vi "QCPFileWrite.vi"(9 "Path Relative?":bool=TRUE, 10 "File Path":string, 11 "QCP Data Block In":T1) -> (0 "error out":errorcluster, 3 "QCP Data Block Out":T1)   [LabVIEW 2015]
uses:
  <userlib>/836-Library/System/QCP Support Code/QCP Data Block.ctl
  <vilib>/Utility/file.llb/Write To Spreadsheet File (string).vi
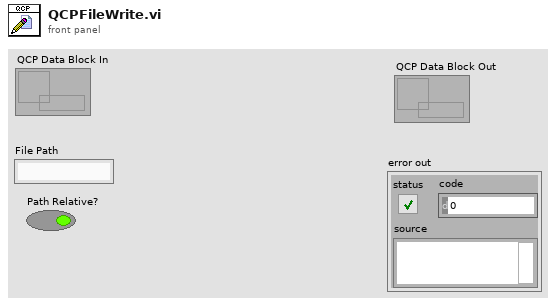
[diagram p1: front panel]
types:
  T1 = typedef "QCP Data Block.ctl" = refnum<data-value>
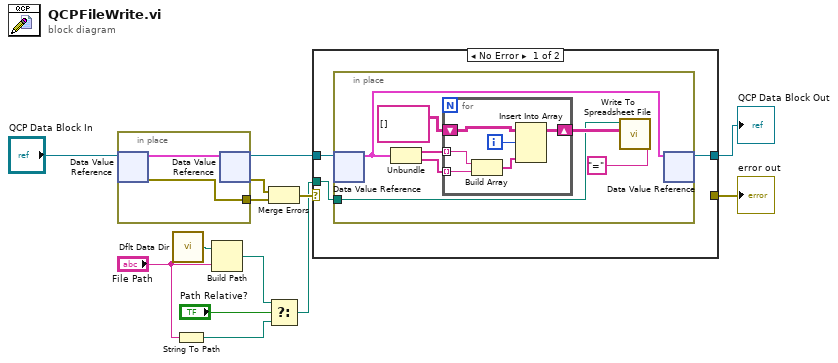
[diagram p0: block diagram]
diagram:
  n1 = in-place {
    in-place-border: [w14] -> w12
    n2 = in-place-dvr #1("QCP Data Block In") -> (w15:cluster{string[], string[]}, w14:errorcluster)
    n3 = in-place-dvr #1(w15) -> (w10:T1, w13:errorcluster)
  }
  n4 = call <vilib>:"Dflt Data Dir.vi"() -> ("App:Default Data Directory"=w1:path)
  n5 = String To Path(string="File Path") -> (path=w3:path)
  n6 = Build Path(base path=w1, name or relative path="File Path") -> (appended path=w2:path)
  n7 = Merge Errors(w13, w12) -> (w11:errorcluster)
  n8 = Select(t=w2, s="Path Relative?", f=w3) -> (s? t:f=w5:path)
  n9 = case shown="No Error" w11 {
    selector: w11 -> [_ w32]
    tunnel: [w18 w33] -> w9
    tunnel: w10 -> [w17 w33]
    tunnel: w5 -> [w16 _]
    tunnel: [_ w32] -> w7
    frame No Error {
      n10 = in-place {
        in-place-border: w16 -> [w21]
        n11 = in-place-dvr #2(w17) -> (w19:cluster{string[], string[]})  [unwired: 1 out]
        n12 = Unbundle(w19) -> (w25:string[], w24:string[])
        n13 = for {
          tunnel: w25 -> [w30] mode=indexing
          tunnel: w24 -> [w29] mode=indexing
          shift-right: [w26] -> w22
          shift-left: string[][] [] ("initialized array") -> [w27]
          i -> [w31]
          n14 = Build Array(w30, w29) -> (w28:string[])
          n15 = Insert Into Array(array=w27, index (row)=w31, new element=w28) -> (w26:string[][])  [unwired: 1 in]
        }
        n16 = call-poly <vilib>:"Write To Spreadsheet File.vi"("delimiter (\\t)"="=" ("delimiter (\\t)"), "2D data"=w22, "file path (dialog if empty)"=w21) -> ()  [unwired: 5 in, 1 out]
        n17 = in-place-dvr #2(w19) -> (w18:T1)  [unwired: 1 out]
      }
    }
    frame Error {
    }
  }
  "QCP Data Block Out" <- w9
  "error out" <- w7
